vi "HTS_INITIALIZE.vi"(6 "Error IN":errorcluster, 9 "VISA resource IN":refnum<visa-resource-name>="HTS") -> (0 "Error OUT":errorcluster, 3 "VISA resource OUT":refnum<visa-resource-name>)   [LabVIEW 2013]
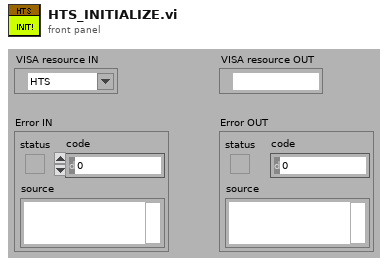
[diagram p1: front panel]
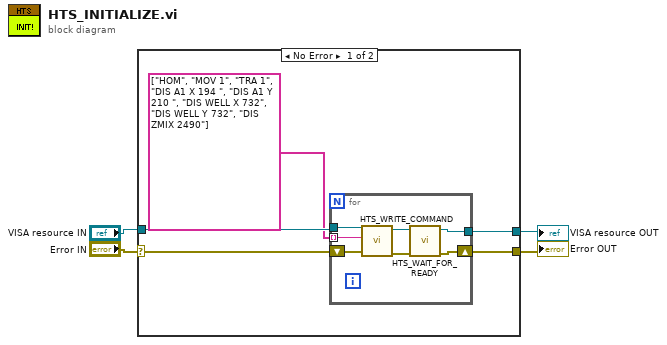
[diagram p0: block diagram]
diagram:
  n1 = case shown="No Error" "Error IN" {
    selector: "Error IN" -> [w6 w17]
    tunnel: [w9 w18] -> w4
    tunnel: [w8 w17] -> w3
    tunnel: "VISA resource IN" -> [w7 w18]
    frame No Error {
      n2 = for {
        tunnel: [w16] -> w9
        tunnel: w7 -> [w12]
        shift-right: [w15] -> w8
        shift-left: w6 -> [w11]
        tunnel: string[] ["HOM", "MOV 1", "TRA 1", "DIS A1 X 194 ", "DIS A1 Y 210 ", "DIS WELL X 732", "DIS WELL Y 732", "DIS ZMIX 2490"] -> [w10] mode=indexing
        n3 = call "HTS_WRITE_COMMAND.vi"("Error IN"=w11, "Command"=w10, "VISA resource IN"=w12) -> ("Error OUT"=w13:errorcluster, "VISA resource OUT"=w14:refnum<visa-resource-name>)  [unwired: 7 out]
        n4 = call "HTS_WAIT_FOR_READY.vi"("Error IN"=w13, "VISA resource IN"=w14) -> ("Error OUT"=w15:errorcluster, "VISA resource OUT"=w16:refnum<visa-resource-name>)  [unwired: 1 in, 7 out]
      }
    }
    frame Error {
    }
  }
  "VISA resource OUT" <- w4
  "Error OUT" <- w3
